vi "QTrkSelectDLLDialog.vi"(9 "Just set path, don't show dialog (F)":bool, 10 "cuda?":bool, 11 "Use debug library":bool) -> (3 "Output":path)   [LabVIEW 2011]
uses:
  QTrkDLL.vi
panel:
  in  "stop":bool
  in  "Tab Control":enum32{"Standard path", "Explicit path "}(tab)
  out "Resulting path":path
  in  "Use development path":bool
  in  "Select path":path
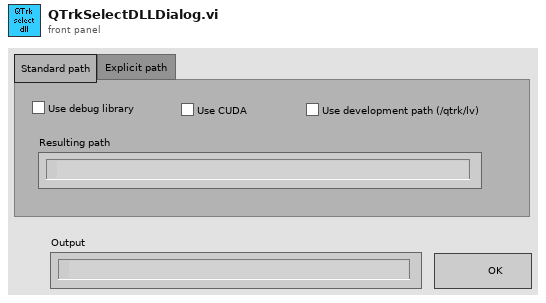
[diagram p1: front panel]
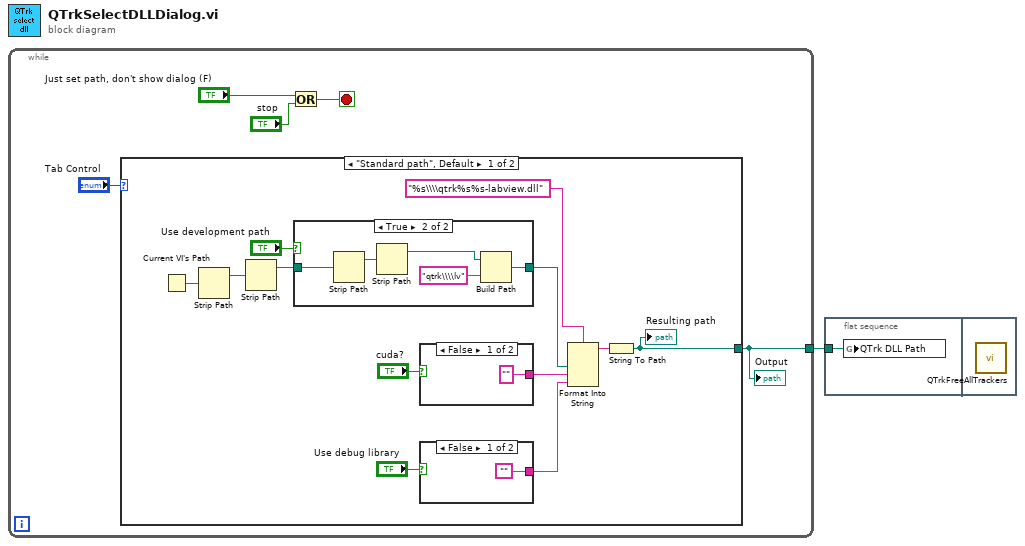
[diagram p0: block diagram]
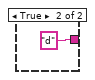
[diagram p3: hidden frame]
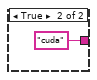
[diagram p4: hidden frame]
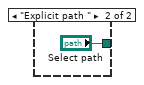
[diagram p5: hidden frame]
diagram:
  n1 = while {
    tunnel: [w5] -> w1
    stop <- w2 stop-if-true
    n2 = case shown="\"Standard path\", Default" "Tab Control" {
      tunnel: [w12 "Select path"] -> w5
      frame "Standard path", Default {
        n3 = Current VI's Path() -> (path=w11:path)
        n4 = Strip Path(path=w11) -> (stripped path=w10:path)  [unwired: 1 out]
        n5 = Strip Path(path=w10) -> (stripped path=w9:path)  [unwired: 1 out]
        n6 = case shown="True" "Use development path" {
          tunnel: w9 -> [w19 w24]
          tunnel: [w19 w22] -> w7
          frame False {
          }
          frame True {
            n7 = Strip Path(path=w24) -> (stripped path=w21:path)  [unwired: 1 out]
            n8 = Strip Path(path=w21) -> (stripped path=w20:path)  [unwired: 1 out]
            n9 = Build Path(base path=w20, name or relative path="qtrk\\\\lv") -> (appended path=w22:path)
          }
        }
        n10 = case shown="False" "cuda?" {
          tunnel: ["" "cuda"] -> w15
          frame False {
          }
          frame True {
          }
        }
        n11 = case shown="False" "Use debug library" {
          tunnel: ["" "d"] -> w14
          frame False {
          }
          frame True {
          }
        }
        n12 = Format Into String(format string="%s\\\\qtrk%s%s-labview.dll", w7, w15, w14) -> (resulting string=w13:string)  [unwired: 2 in, 1 out]
        n13 = String To Path(string=w13) -> (path=w12:path)
        "Resulting path" <- w12
      }
      frame "Explicit path " {
      }
    }
    "Output" <- w5
    n14 = Or(x="Just set path, don't show dialog (F)", y="stop") -> (x .or. y?=w2:bool)
  }
  n15 = flat-sequence {
    tunnel: w1 -> [w30]
    frame #0 {
      n16 = global write "QTrkDLL.vi" "QTrk DLL Path"(w30) -> ()
    }
    frame #1 {
      n17 = call "QTrkFreeAllTrackers.vi"() -> ()  [unwired: 12 in]
    }
  }
